vi "Start.vi"(8 "error in (no error)":errorcluster, 10 "Message in":refnum<class "StartMessage.lvclass">, 11 "Thorcam in":refnum<class "Thorcam.lvclass">) -> (0 "error out":errorcluster, 3 "Thorcam out":refnum<class "Thorcam.lvclass">)   [LabVIEW 2012, in "Thorcam.lvclass"]
doc: "This member function is called when the statemachine in the run.vi receives an 'start' command. It relays the message to all observers of the component.\n\nOverride this member function in your derived class if you need additional start functionality (but don't forget to call the parent method)."
uses:
  Thorcam.lvclass
  <vilib>/Distrio/Murmex/Murmex/Murmex.lvclass
  <vilib>/Distrio/Murmex/StartMessage/StartMessage.lvclass
  imaging mode.ctl
  <vilib>/Distrio/Murmex/ProceedMessage/ProceedMessage.lvclass
  <vilib>/Distrio/Murmex/GenericMessage/GenericMessage.lvclass
panel:
  # "This member function is called when the statemachine in the run.vi receives an 'start' command. It relays the message to all observers of the component.\n\nOverride this member function in your derived class if you need additional start functionality (but don't forget to call the parent method)."
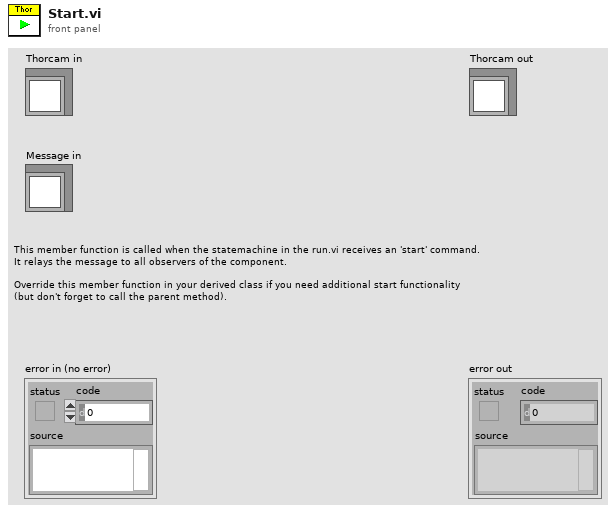
[diagram p1: front panel]
types:
  T1 = typedef "Thorcam.lvclass/imaging mode.ctl" = enum16{"free run mode", "single frame"}
  T2 = typedef "Murmex.lvlib/StartMessage.lvclass/run mode enum.ctl" = enum16{"infinite", "finite"}
  T3 = typedef "Thorcam.lvclass/current task.ctl" = enum16{"Camera", "Phase Comparison", "Pre-Tomo"}
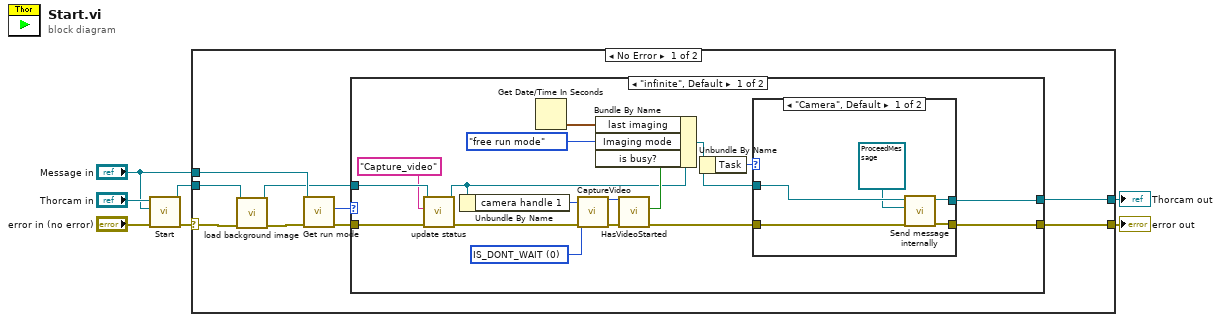
[diagram p0: block diagram]
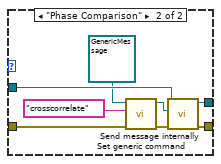
[diagram p2: hidden frame]
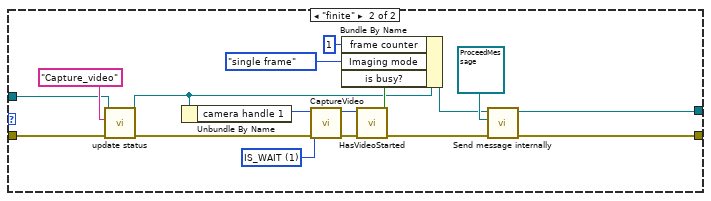
[diagram p3: hidden frame]
diagram:
  n1 = call-parent "Start.vi"("error in (no error)"="error in (no error)", "Message in"="Message in", "Murmex in"="Thorcam in") -> ("error out"=w5:errorcluster, "Murmex out"=w3:refnum<class "Thorcam.lvclass">)  [unwired: 7 in]
  n2 = case shown="No Error" w5 {
    selector: w5 -> [w11 w65]
    tunnel: [w16 w65] -> w4
    tunnel: w3 -> [w9 w64]
    tunnel: [w15 w64] -> w2
    tunnel: "Message in" -> [w14 _]
    frame No Error {
      n3 = call-dynamic "load background image.vi"("error in (no error)"=w11, "Thorcam in"=w9) -> ("error out"=w10:errorcluster, "Thorcam out"=w8:refnum<class "Thorcam.lvclass">)  [unwired: 8 in]
      n4 = call <vilib>:"Get run mode.vi"("error in (no error)"=w10, "StartMessage in"=w14) -> ("error out"=w12:errorcluster, "run mode"=w13:T2)  [unwired: 7 in, 1 out]
      n5 = case shown="\"infinite\", Default" w13 {
        tunnel: [w19 w48] -> w16
        tunnel: [w20 w49] -> w15
        tunnel: w12 -> [w25 w53]
        tunnel: w8 -> [w23 w51]
        frame "infinite", Default {
          w18 = 0 items=["IS_DONT_WAIT", "IS_WAIT"] ("Wait")
          n6 = call-dynamic "update status.vi"("error in (no error)"=w25, "status in"="Capture_video", "Thorcam in"=w23) -> ("error out"=w24:errorcluster, "Thorcam out"=w22:refnum<class "Thorcam.lvclass">)  [unwired: 7 in]
          n7 = Unbundle By Name(w22) -> ("camera handle 1"=w33:u32)
          n8 = Get Date/Time In Seconds() -> (seconds since 1Jan1904=w17:timestamp)
          n9 = call <instrlib>:"CaptureVideo.vi"("error in"=w24, "Wait"=w18, "Camera Handle In"=w33) -> ("error out"=w32:errorcluster, "Camera Handle Out"=w31:u32)  [unwired: 7 in]
          n10 = call <instrlib>:"HasVideoStarted.vi"("error in"=w32, "Camera Handle In"=w31) -> ("error out"=w28:errorcluster, "Video started"=w30:bool)  [unwired: 7 in, 1 out]
          n11 = Bundle By Name(cluster=w22, "last imaging"=w17, "Imaging mode"=imaging_mode."free run mode", "is busy?"=w30) -> (w27:refnum<class "Thorcam.lvclass">)
          n12 = Unbundle By Name(w27) -> ("Task"=w26:T3)
          n13 = case shown="\"Camera\", Default" w26 {
            tunnel: w28 -> [w37 w43]
            tunnel: w27 -> [w36 w42]
            tunnel: [w35 w40] -> w20
            tunnel: [w38 w39] -> w19
            frame "Camera", Default {
              n14 = call <vilib>:"Send message internally.vi"("error in (no error)"=w37, "Message"=refnum<class "ProceedMessage.lvclass"> refnum ("Distrio Murmex 1.5:ProceedMessage"), "Murmex in"=w36) -> ("error out"=w38:errorcluster, "Murmex out"=w35:refnum<class "Thorcam.lvclass">)  [unwired: 7 in]
            }
            frame "Phase Comparison" {
              n15 = call <vilib>:"Set generic command.vi"("error in (no error)"=w43, "generic command"="crosscorrelate", "GenericMessage in"=refnum<class "GenericMessage.lvclass"> refnum ("Distrio Murmex 1.1:GenericMessage")) -> ("error out"=w45:errorcluster, "GenericMessage out"=w44:refnum<class "GenericMessage.lvclass">)  [unwired: 7 in]
              n16 = call <vilib>:"Send message internally.vi"("error in (no error)"=w45, "Message"=w44, "Murmex in"=w42) -> ("error out"=w39:errorcluster, "Murmex out"=w40:refnum<class "Thorcam.lvclass">)  [unwired: 7 in]
            }
          }
        }
        frame "finite" {
          w47 = 1 items=["IS_DONT_WAIT", "IS_WAIT"] ("Wait")
          n17 = call-dynamic "update status.vi"("error in (no error)"=w53, "status in"="Capture_video", "Thorcam in"=w51) -> ("error out"=w52:errorcluster, "Thorcam out"=w50:refnum<class "Thorcam.lvclass">)  [unwired: 7 in]
          n18 = Unbundle By Name(w50) -> ("camera handle 1"=w63:u32)
          n19 = call <instrlib>:"CaptureVideo.vi"("error in"=w52, "Wait"=w47, "Camera Handle In"=w63) -> ("error out"=w60:errorcluster, "Camera Handle Out"=w61:u32)  [unwired: 7 in]
          n20 = call <instrlib>:"HasVideoStarted.vi"("error in"=w60, "Camera Handle In"=w61) -> ("error out"=w56:errorcluster, "Video started"=w59:bool)  [unwired: 7 in, 1 out]
          n21 = Bundle By Name(cluster=w50, "frame counter"=1 ("runtime.frame counter"), "Imaging mode"=imaging_mode."single frame", "is busy?"=w59) -> (w55:refnum<class "Thorcam.lvclass">)
          n22 = call <vilib>:"Send message internally.vi"("error in (no error)"=w56, "Message"=refnum<class "ProceedMessage.lvclass"> refnum ("ProceedMessage"), "Murmex in"=w55) -> ("error out"=w48:errorcluster, "Murmex out"=w49:refnum<class "Thorcam.lvclass">)  [unwired: 7 in]
        }
      }
    }
    frame Error {
    }
  }
  "error out" <- w4
  "Thorcam out" <- w2
